vi "1-FindActor.vi"(3 "ProjectIndex":i32) -> (0 "Actors":refnum<vi>[][](array[refnum]), 1 "Project-Name":string)   [LabVIEW 2016, in "TestVIs.lvlib"]
uses:
  TestVIs.lvlib
panel:
  out "Actors":string[][](array[string])
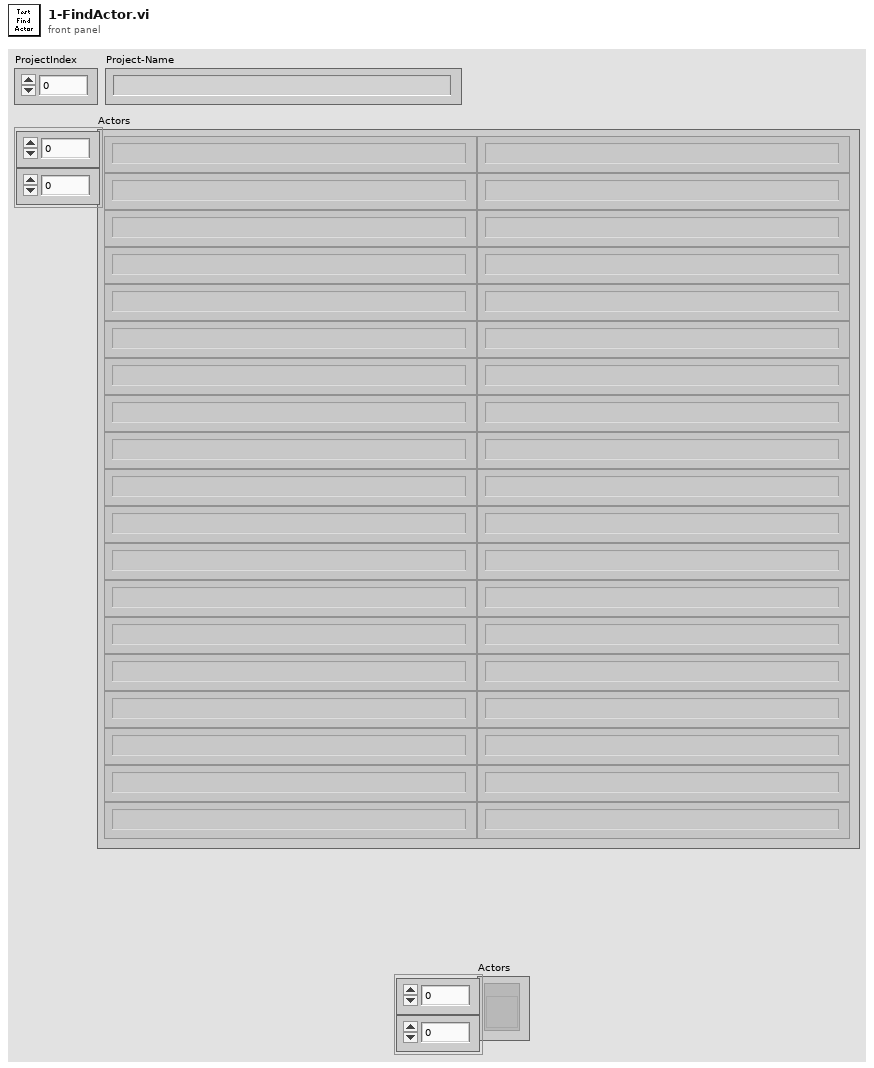
[diagram p1: front panel]
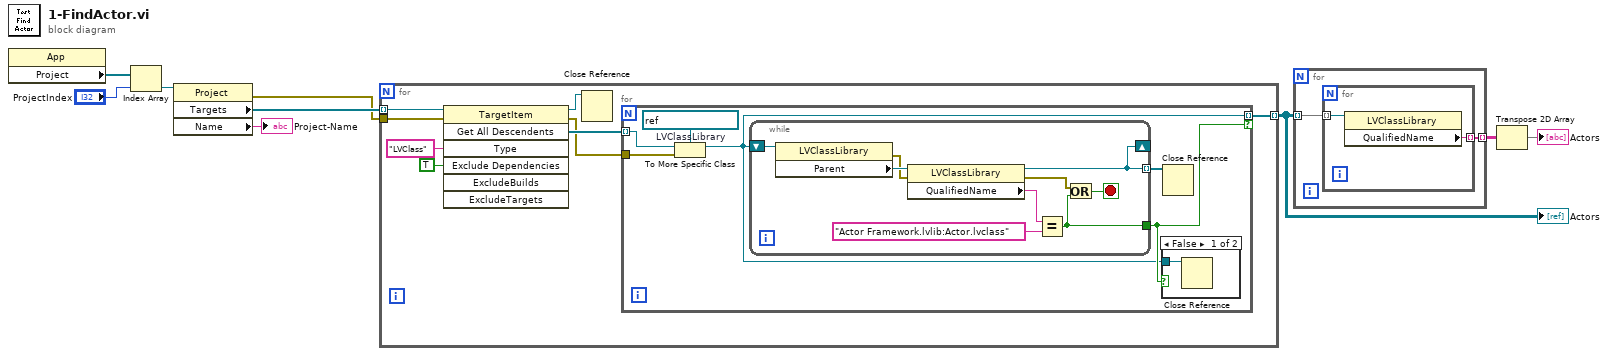
[diagram p0: block diagram]
diagram:
  n1 = property class="App"() -> ("Project"=w7:refnum<vi>[])  [unwired: 2 in, 2 out]
  n2 = Index Array(array=w7, index="ProjectIndex") -> (element=w6:refnum<vi>)
  n3 = property class="Project"(reference=w6) -> (error out=w8:errorcluster, "Targets"=w9:refnum<vi>[], "Name"=→"Project-Name":string)  [unwired: 1 in, 1 out]
  n4 = for {
    tunnel: w9 -> [w16] mode=indexing
    tunnel: w8 -> [w15]
    tunnel: [w10] -> w2 mode=indexing
    n5 = invoke class="TargetItem" method="Get All Descendents"(reference=w16, error in=w15, "Type"="LVClass", "Exclude Dependencies"=TRUE ("ExcludeDependencies")) -> (reference out=w12:refnum<vi>, error out=w11:errorcluster, "All Descendents"=w13:refnum<vi>[])  [unwired: 3 in, 4 out]
    n6 = Close Reference(reference=w12) -> ()  [unwired: 1 in, 1 out]
    n7 = for {
      tunnel: w13 -> [w22] mode=indexing
      tunnel: w11 -> [w21]
      tunnel: [w18] -> w10 mode=indexing if=w19
      w23 = refnum<vi> refnum  # LVClassLibrary
      n8 = To More Specific Class(target class=w23, reference=w22, error in=w21) -> (specific class reference=w18:refnum<vi>)  [unwired: 1 out]
      n9 = while {
        shift-right: [w27] -> _
        shift-left: w18 -> [w33]
        tunnel: [w27] -> w20 mode=indexing
        tunnel: [w26] -> w19
        stop <- w28 stop-if-true
        n10 = property class="LVClassLibrary"(reference=w33) -> (error out=w25:errorcluster, "Parent"=w29:refnum<vi>)  [unwired: 1 in, 1 out]
        n11 = property class="LVClassLibrary"(reference=w29, error in=w25) -> (reference out=w27:refnum<vi>, error out=w30:errorcluster, "QualifiedName"=w32:string)
        n12 = Equal?(x=w32, y="Actor Framework.lvlib:Actor.lvclass") -> (x = y?=w26:bool)
        n13 = Or(x=w30, y=w26) -> (x .or. y?=w28:bool)
      }
      n14 = case shown="False" w19 {
        tunnel: w18 -> [w24 _]
        frame False {
          n15 = Close Reference(reference=w24) -> ()  [unwired: 1 in, 1 out]
        }
        frame True {
        }
      }
      n16 = Close Reference(reference=w20) -> ()  [unwired: 1 in, 1 out]
    }
  }
  "Actors" <- w2
  n17 = for {
    tunnel: w2 -> [w35] mode=indexing
    tunnel: [w34] -> w5 mode=indexing
    n18 = for {
      tunnel: w35 -> [w37] mode=indexing
      tunnel: [w36] -> w34 mode=indexing
      n19 = property class="LVClassLibrary"(reference=w37) -> ("QualifiedName"=w36:string)  [unwired: 1 in, 2 out]
    }
  }
  n20 = Transpose 2D Array(2D array=w5) -> (transposed array=→"Actors":string[][])
